vi "ArmSoftLimitChecks.vi"() -> ()   [LabVIEW 2020]
panel:
  in  "Encoder Max":dbl format="%#_13g"
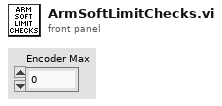
[diagram p1: front panel]
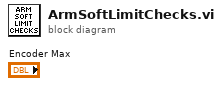
[diagram p0: block diagram]
diagram:
